vi "tanh.vi"(6 "label":T1, 8 "error in (no error)":errorcluster, 11 "A":refnum<class "Value.lvclass">) -> (0 "error out":errorcluster, 2 "C":refnum<class "Value.lvclass">, 3 "A out":refnum<class "Value.lvclass">)   [LabVIEW 2023, in "LabGRAD.lvlib" / "Value.lvclass"]
uses:
  Value.lvclass
  UiObjects/string control.ctl
  operation.ctl
  Value.lvclass/Value.ctl
  UiObjects/UiObjects.lvclass
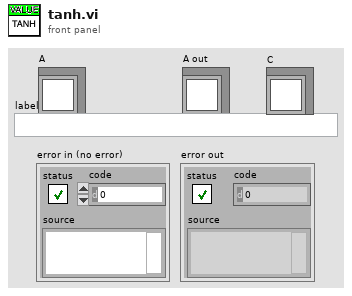
[diagram p1: front panel]
types:
  T1 = typedef "UiObjects.lvlib/UiObjects.lvclass/string control.ctl" = string
  T2 = typedef "LabGRAD.lvlib/Value.lvclass/operation.ctl" = enum16{"nop", "add", "subtract", "power", "multiply", "divide", "tanh"}
  T3 = typedef "UiObjects.lvlib/UiObjects.lvclass/numeric value control.ctl" = dbl
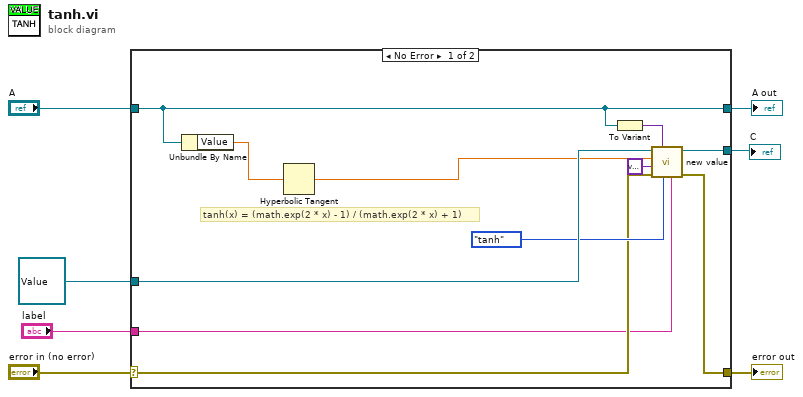
[diagram p0: block diagram]
diagram:
  n1 = case shown="No Error" "error in (no error)" {
    selector: "error in (no error)" -> [w13 w21]
    tunnel: [w12 w21] -> w6
    tunnel: [w16 w20] -> w4
    tunnel: "A" -> [w16 w20]
    tunnel: refnum<class "Value.lvclass"> refnum ("B") -> [w18 w19]
    tunnel: [w17 w19] -> w2
    tunnel: "label" -> [w11 _]
    frame No Error {
      # "tanh(x) = (math.exp(2 * x) - 1) / (math.exp(2 * x) + 1)"
      n2 = Unbundle By Name(w16) -> ("Value"=w9:T3)
      n3 = Hyperbolic Tangent(1:w9) -> (0:w8:T3)
      n4 = To Variant(anything=w16) -> (Variant=w15:variant)
      n5 = call "new value.vi"("Label"=w11, "operation"=operation."tanh", "Previous"=w15, "error in (no error)"=w13, "Other"=variant, "data"=w8, "Value in"=w18) -> ("error out"=w12:errorcluster, "Value out"=w17:refnum<class "Value.lvclass">)  [unwired: 3 in]
    }
    frame Error {
    }
  }
  "error out" <- w6
  "A out" <- w4
  "C" <- w2
